vi "AOD Control (FPGA).vi"() -> ()   [LabVIEW 2011]
uses:
  FPGAState.ctl
  AODCalibration.ctl
  CoordinateSettings.ctl
  <vilib>/Platform/TimedLoop/XDataNode/timing_clust.ctl
  <vilib>/Platform/TimedLoop/XDataNode/nitl_modes.ctl
  <vilib>/Platform/TimedLoop/XDataNode/wakeup.ctl
  <vilib>/rvi/eio/common/nirviEmuTemplateMethod_errors.vi
  <vilib>/rvi/interface/RandomDataEmulation/nirviRandomDataFPGAFIFO.vi
  <vilib>/rvi/interface/RandomDataEmulation/niFpgaRandomDataHandleErrors.vi
  <vilib>/Platform/TimedLoop/XDataNode/XDataNode.xnode
  <vilib>/eio/EIONode/EIONode.xnode
  <vilib>/rvi/DataTransferAndStorage/Container/XNode/niFpgaContainer.xnode
  <vilib>/rvi/interface/RandomDataEmulation/nirviRandomDataFpgaReadWriteTemplate.vi
  <vilib>/Platform/TimedLoop/XDataNode/XDNodeRunTimeDep.lvlib
panel:
  out "Debug.Settings":T1 {"YLP_RR" format="%x"; "YLP_FR" format="%x"; "YHP_RR" format="%x"; "YHP_FR" format="%x"; "XLP_RR" format="%x"; "XLP_FR" format="%x"; "XHPstart" format="%x"; "XHPend" format="%x"; "XLPstart" format="%x"; "XLPend" format="%x"; "YHPstart" format="%x"; "YHPend" format="%x"; "YLPstart" format="%x"; "YLPend" format="%x"; "XHP_RR" format="%x"; "XHP_FR" format="%x"}
  out "Raw Full":bool
  in  "Setup.Stop on full":bool
  in  "Setup.BitShift":i16=-10
  in  "Setup.Downsample":u32=1000
  out "Status.Update IO Missing":bool
  out "Status.Last Point":bool
  out "Status.All Samples":bool
  out "Status.Serial error":bool
  out "Status.AcqState":enum16{"Idling", "Acquiring"}(ring)
  out "Status.TemporalChFull":bool
  out "Status.MotionChFull":bool
  out "Status.DownsampleDone":bool
  out "Status.ImChFull":bool
  out "Status.BufferedPoints":i32
  out "Status.State":T2
  out "Status.Initialized":bool
  out "Status.RepNum":u32
  out "Status.OutOfRange":bool
  out "Status.Mode":enum16{"Points", "Volume", "Idle"}(ring)
  out "Status.ScanDone":bool
  out "Status.Armed":bool
  out "Status.ScanUpdateIO":bool
  out "Status.Writing":bool
  out "Status.PointTime":u32
  out "Status.PointNum":u32
  out "Status.Sequencing error":bool
  out "Analog Data":i16[](array[numeric])
  in  "Update IO timeout":u32=40
  out "UpdateIO counter":u32
  in  "AOD.Calibration":T3={"XHP ChirpGain"=1.0, "YHP ChirpGain"=1.0, "XLP ChirpGain"=1.0, "YLP ChirpGain"=1.0}
  in  "AOD.ThrowawaySamples":u16=40
  in  "AOD.LP Center Frequency":u32=858993459 format="%x"
  in  "AOD.HP Center Frequency":u32=805306367 format="%x"
  in  "AOD.Range":u32=214748364 format="%x"
  in  "AOD.BlankSamples":u16=500
  in  "AOD.UpdatesPerPoint":u32=2000
  out "Downsample Counter":u32
  in  "Scan.NumMotionPoints":u32
  in  "Scan.Motion Increment":u32
  in  "Scan.TotalSamples":u32
  in  "Scan.VolumeSettings":T4={"XStart"=0, "XEnd"=0, "XNum"=1, "YStart"=0, "YEnd"=0, "YNum"=1, "ZStart"=0, "ZEnd"=0, "ZNum"=1} {"ZNum" min=1 max=10000; "YNum" min=1 max=10000; "XNum" min=1 max=10000}
  in  "Scan.NumReps":i32=1
  in  "Scan.NumPoints":u32
  out "Scan.Samples":u32
  out "Debug.PMT_Unpacked_backlog":u32
  out "Debug.PMT_Data_backlog":u32
  in  "Debug.FinishedSettingSize":i16=3
  in  "Debug.FinishedSetting":cluster{"Address":u8, "Value":u32}[](array[cluster])=[{"Address"=0, "Value"=246}, {"Address"=4, "Value"=0}, {"Address"=5, "Value"=0}, {"Address"=0, "Value"=0}, {"Address"=0, "Value"=0}] {"Address" format="%x"; "Value" format="%x"}
  in  "Debug.Coordinate":T5
  in  "Debug.SetCoordinate":bool
  out "Debug.AcqDivCount":u32
  out "Debug.PMT_Samples":u32
  out "Debug.MainLoopCount":i32
  in  "Debug.UpdateIO":bool
  out "Debug.PMT Array":i32[](array[numeric])
  in  "Debug.P":bool
  in  "Debug.Point":cluster{"X":i32, "Y":i32, "Z":i32}
  in  "Debug.Write Point":bool
  in  "Control.Points":bool
  in  "Control.Reset":bool
  in  "Control.Abort":bool
  in  "Control.Volume":bool
  in  "Control.Stop":bool
  in  "Comm.P high":u32=10
  in  "Comm.Pause":u32
  in  "Comm.WriteSize":i32
  in  "Comm.Write":cluster{"Address":u8, "Value":u32}[](array[cluster])=[{"Address"=0, "Value"=0}, {"Address"=0, "Value"=0}, {"Address"=0, "Value"=0}, {"Address"=0, "Value"=0}, {"Address"=0, "Value"=0}, {"Address"=0, "Value"=0}, {"Address"=0, "Value"=0}, {"Address"=0, "Value"=0}, {"Address"=0, "Value"=0}, {"Address"=0, "Value"=0}, {"Address"=0, "Value"=0}, {"Address"=0, "Value"=0}, {"Address"=0, "Value"=0}, {"Address"=0, "Value"=0}, {"Address"=0, "Value"=0}, {"Address"=0, "Value"=0}, {"Address"=0, "Value"=0}, {"Address"=0, "Value"=0}, {"Address"=0, "Value"=0}, {"Address"=0, "Value"=0}]
  out "Comm.Written":cluster{"Address":u8, "Value":u32}[](array[cluster])
  out "Comm.WritenCount":i32
  in  "Comm.Write Register":bool
  in  "Comm.SclkDivider":u32=10
  in  "Comm.CommLines":enum16{"1", "2", "4"}(ring)
  out "Comm.Bad Coordinate":bool
  in  "Comm.UpdateIO time":u32=2
  # "TriggerAcq makes this task\n require a trigger from Trig7"
  # "FPGA Control state chart:\n1. Idles\n2. Write series of registers\n3. Receive volume settings or points, \n    arms task, starts  acq clock.  \n4. Clock in first value, waits for Trig7\n5. On Trig7 pulse start task\n6. Pulse update_io, clock point, count\n    downsample number of acq clocks"
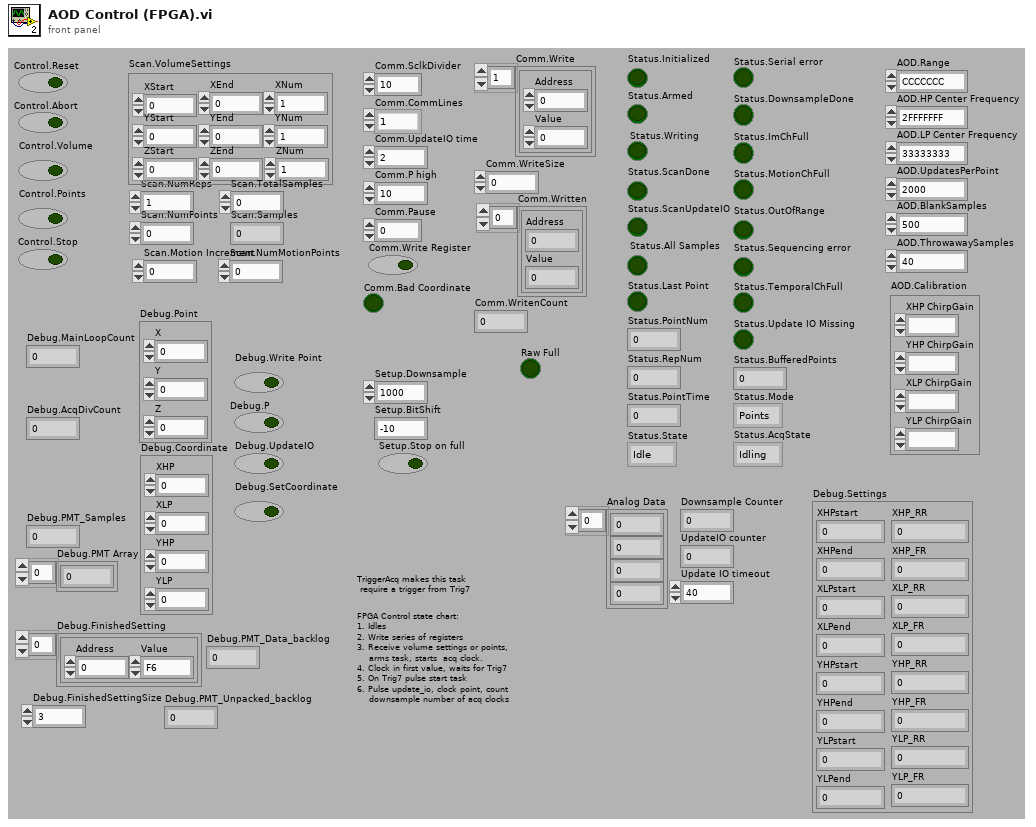
[diagram p1: front panel]
types:
  T1 = typedef "CoordinateSettings.ctl" = cluster{"XHPstart":u32, "XHPend":u32, "XLPstart":u32, "XLPend":u32, "YHPstart":u32, "YHPend":u32, "YLPstart":u32, "YLPend":u32, "XHP_RR":u32, "XHP_FR":u32, "XLP_FR":u32, "XLP_RR":u32, "YHP_FR":u32, "YHP_RR":u32, "YLP_FR":u32, "YLP_RR":u32}
  T2 = typedef "FPGAState.ctl" = enum16{"Idle", "Arm Scan", "Scan", "End Scan"}
  T3 = typedef "AODCalibration.ctl" = cluster{"XHP ChirpGain":fxp<+/-,16,2>, "YHP ChirpGain":fxp<+/-,16,2>, "XLP ChirpGain":fxp<+/-,16,2>, "YLP ChirpGain":fxp<+/-,16,2>}
  T4 = cluster{"XStart":i32, "XEnd":i32, "XNum":i32, "YStart":i32, "YEnd":i32, "YNum":i32, "ZStart":i32, "ZEnd":i32, "ZNum":i32}
  T5 = cluster{"XHP":i32, "XLP":i32, "YHP":i32, "YLP":i32}
  T6 = cluster{"Scan mode":enum16{"Points", "Volume", "Idle"}, "NumPoints":u32, "NumReps":u32, "Motion Increment":u32, "NumMotionPoints":u32, "VolumeSettings":cluster{"XStart":i32, "XEnd":i32, "XNum":i32, "YStart":i32, "YEnd":i32, "YNum":i32, "ZStart":i32, "ZEnd":i32, "ZNum":i32}}
  T7 = typedef "XDNodeRunTimeDep.lvlib/timing_clust.ctl" = cluster{"Expected End [f-1]":u64, "Actual End [f-1]":u64, "Finished Late? [f-1]":bool, "Expected End [i-1]":u64, "Actual End [i-1]":u64, "Finished Late? [i-1]":bool, "Expected Start [i]":u64, "Actual Start [i]":u64, "Expected Start [f]":u64, "Actual Start [f]":u64, "Source Name":string, "Structure Name":string, "Period":i64, "Deadline":i64, "Offset":i64, "Start":i64, "Priority":i32, "Timeout":i32, "Mode":T8, "Wakeup Reason":T9, "Error":errorcluster, "Source Type":string, "Secondary Source Type":string, "Global End Time":u64, "Global Start Time":u64, "Frame Duration":u64, "Iteration Duration":u64, "Assigned CPU":i32, "I/O Scan Engine Mode":u32}
  T8 = typedef "XDNodeRunTimeDep.lvlib/nitl_modes.ctl" = enum32{"No Change", "Process missed periods, maintain original phase", "Discard missed periods, maintain original phase", "Process missed periods, ignore original phase", "Discard missed periods, ignore original phase"}
  T9 = typedef "XDNodeRunTimeDep.lvlib/wakeup.ctl" = enum32{"Normal", "Aborted", "Asynchronous wakeup", "Timing source error", "Timed loop error", "Timeout"}
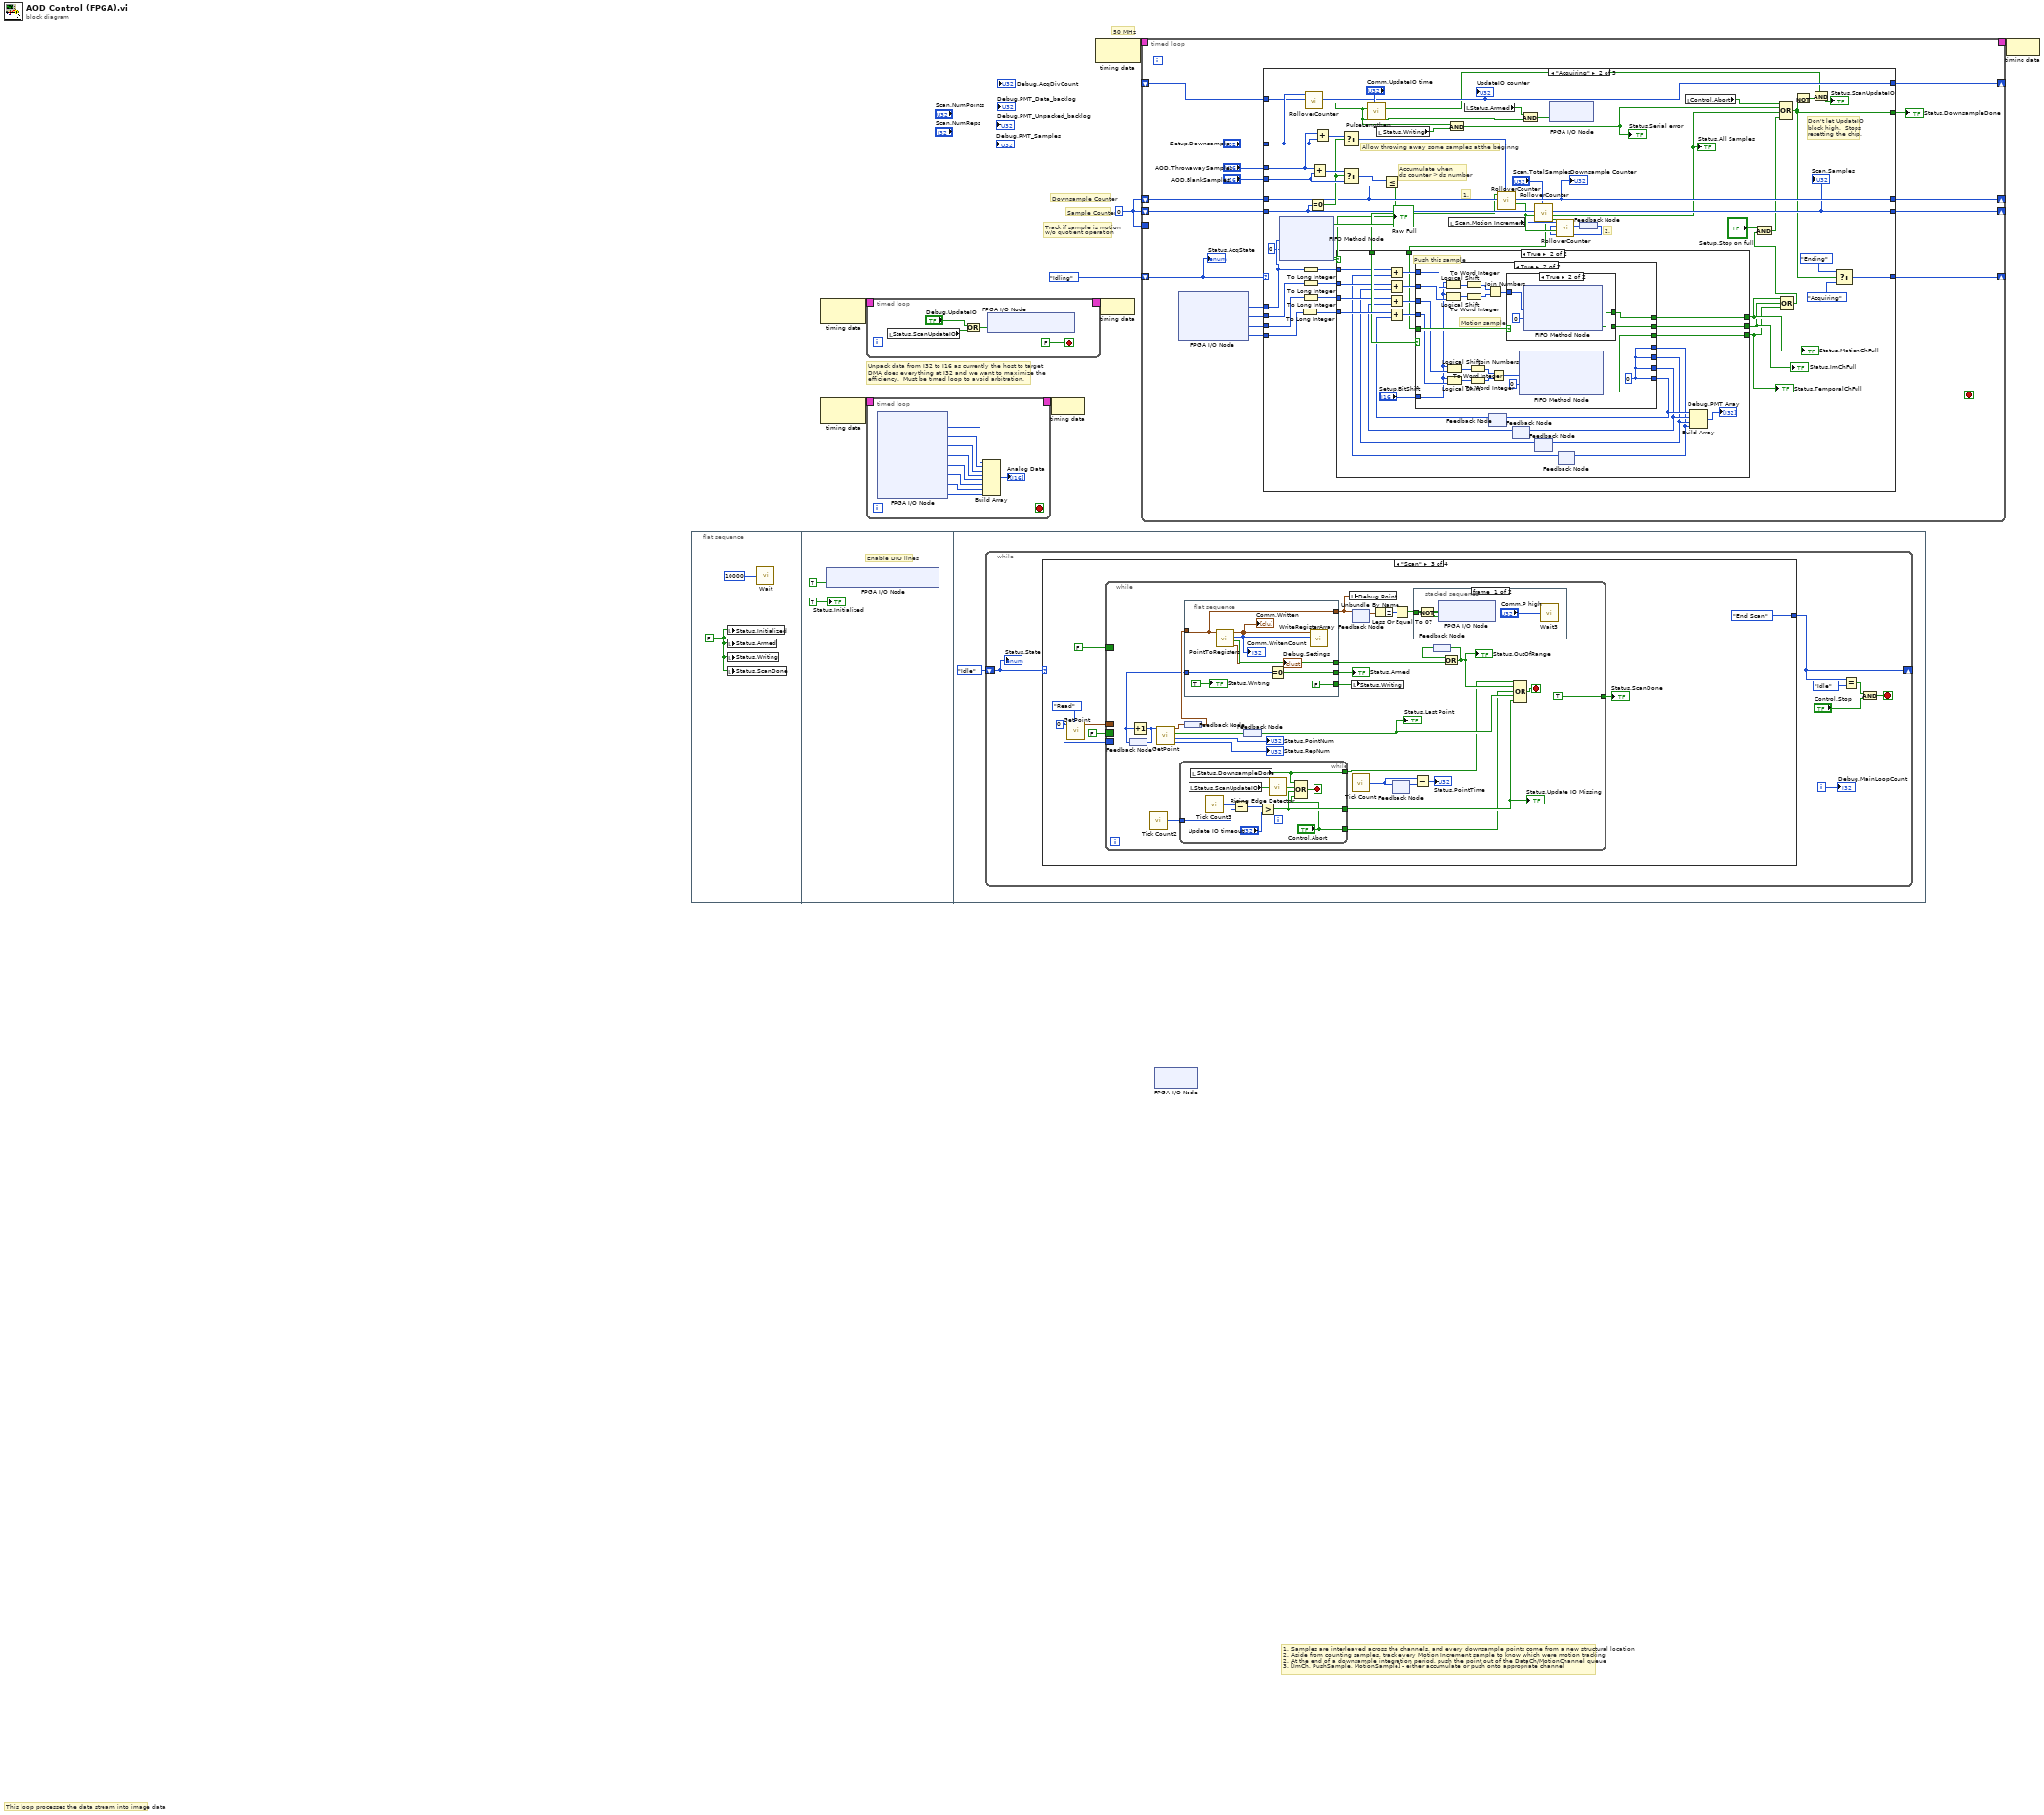
[diagram p0: block diagram]
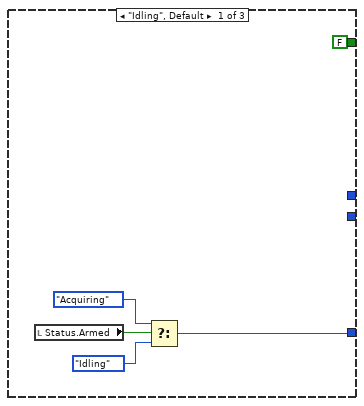
[diagram p2: hidden frame]
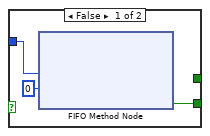
[diagram p5: hidden frame]
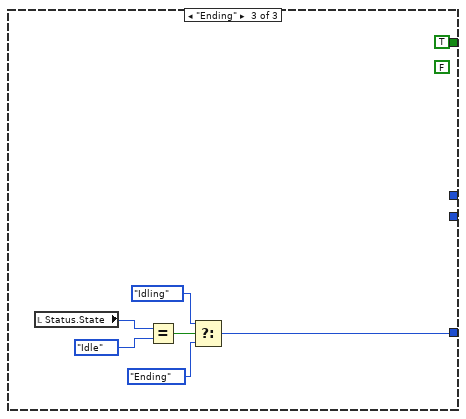
[diagram p6: hidden frame]
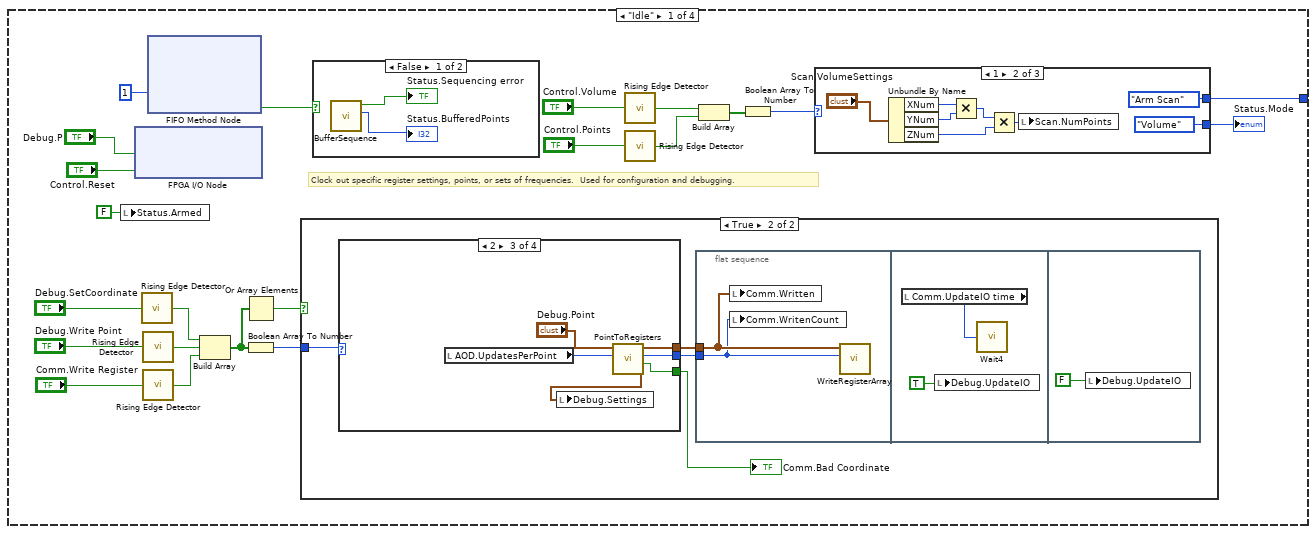
[diagram p7: hidden frame]
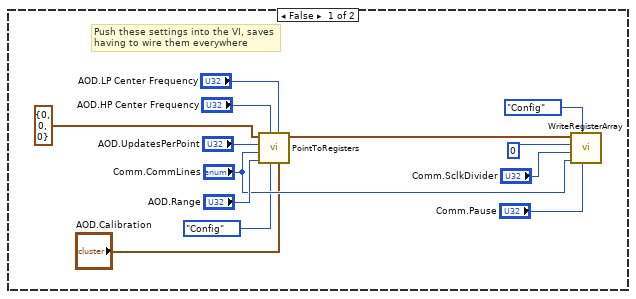
[diagram p9: hidden frame]
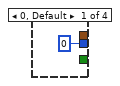
[diagram p10: hidden frame]
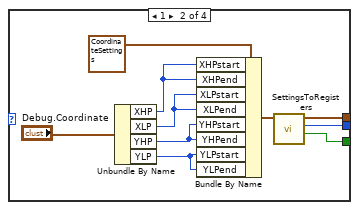
[diagram p11: hidden frame]
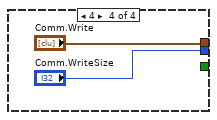
[diagram p12: hidden frame]
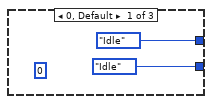
[diagram p13: hidden frame]
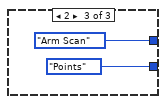
[diagram p14: hidden frame]
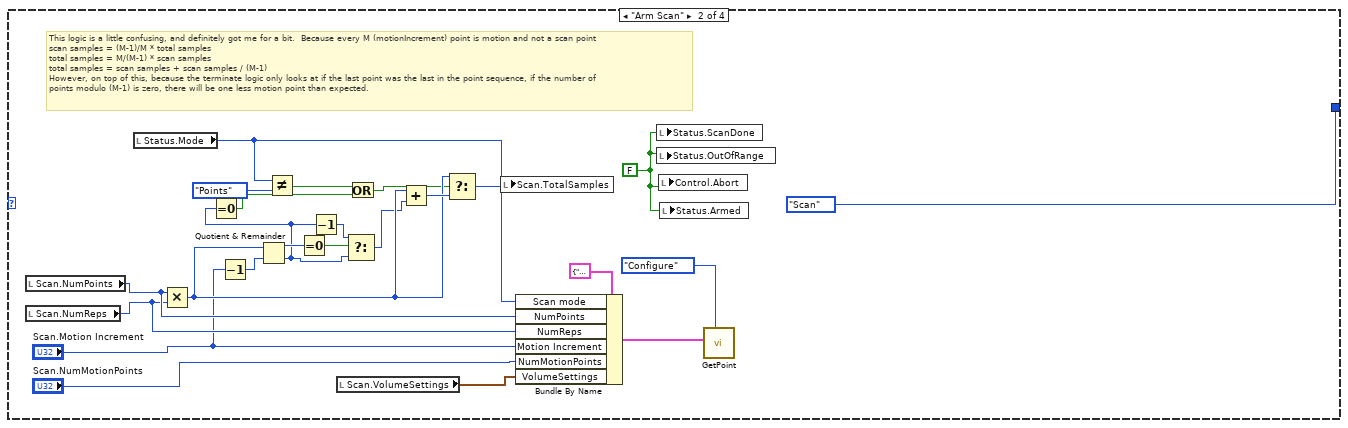
[diagram p15: hidden frame]
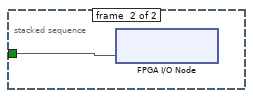
[diagram p16: hidden frame]
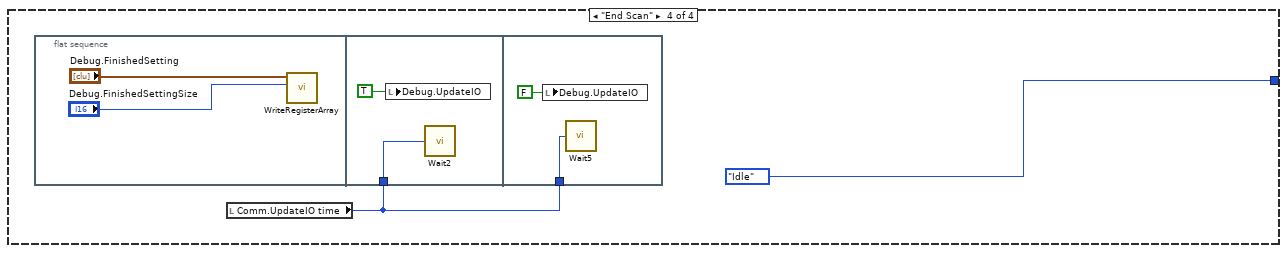
[diagram p17: hidden frame]
diagram:
  w6 = u32 0
  # "Downsample Counter"
  # "Sample Counter"
  # "Track if sample is motion\nw/o quotient operation"
  # "50 MHz"
  # "Unpack data from I32 to I16 as currently the host to target\nDMA does everything at I32 and we want to maximize the\nefficiency.  Must be timed loop to avoid arbitration."
  # "1. Samples are interleaved across the channels, and every downsample points come from a new structural location\n2. Aside from counting samples, track every Motion Increment sample to know which were motion tracking\n2. At the end of a downsample integration period, push the point out of the DataCh/MotionChannel queue\n3. [ImCh, PushSample, MotionSample] - either accumulate or push onto appropriate channel"
  # "This loop processes the data stream into image data"
  n1 = flat-sequence {
    frame #0 {
      w9 = FALSE
      n2 = local write "Status.Initialized"(w9) -> ()
      n3 = local write "Status.Armed"(w9) -> ()
      n4 = local write "Status.Writing"(w9) -> ()
      n5 = local write "Status.ScanDone"(w9) -> ()
      n6 = call "Wait"("Count(uSec)"=u32 10000) -> ()  [unwired: 1 out]
    }
    frame #1 {
      # "Enable DIO lines"
      n7 = xnode "FPGA I/O Node"("IO Module\\Digital Output Enable"=TRUE ("IO Module\\DDCA_DIO0-7_WE")) -> ()  [unwired: 1 in, 1 out]
      "Status.Initialized" <- TRUE ("Status.Initialized")
    }
    frame #2 {
      n8 = while {
        shift-right: [w19] -> _
        shift-left: FPGAState."Idle" ("Ring") -> [w14]
        i -> [w20]
        stop <- w16 stop-if-true
        n9 = case shown="\"Scan\"" w14 {
          tunnel: [w41 FPGAState."Scan" ("Ring") FPGAState."End Scan" ("Ring") FPGAState."Idle" ("Enum")] -> w19
          frame "Idle" {
            # "Clock out specific register settings, points, or sets of frequencies.  Used for configuration and debugging."
            n10 = local write "Status.Armed"(FALSE ("Status.Armed")) -> ()
            n11 = xnode "FPGA I/O Node"("IO Module\\P"="Debug.P", "IO Module\\RESET"="Control.Reset") -> ()  [unwired: 2 in, 2 out]
            n12 = call "Rising Edge Detector.vi"("Signal In"="Debug.SetCoordinate") -> ("Edge Detected?"=w34:bool)
            n13 = call "Rising Edge Detector.vi"("Signal In"="Debug.Write Point") -> ("Edge Detected?"=w33:bool)
            n14 = call "Rising Edge Detector.vi"("Signal In"="Comm.Write Register") -> ("Edge Detected?"=w28:bool)
            n15 = xnode ("FIFO Method Node")("Timeout"=1) -> ("Timed Out?"=w27:bool)  [unwired: 1 in, 2 out]
            n16 = Build Array(w34, w33, w28) -> (w32:bool[])
            n17 = Or Array Elements(Boolean array=w32) -> (logical OR=w31:bool)
            n18 = Boolean Array To Number(Boolean array=w32) -> (number=w30:u8)
            n19 = case shown="True" w31 {
              tunnel: w30 -> [_ w61]
              frame False {
                # "Push these settings into the VI, saves \nhaving to wire them everywhere"
                n20 = call "PointToRegisters.vi"("Calibration"="AOD.Calibration", "LP Center Frequency"="AOD.LP Center Frequency", "Mode"=enum16{"Normal", "Config"}."Config", "HP Center Frequency"="AOD.HP Center Frequency", "Range"="AOD.Range", "WriteSize"="Comm.CommLines", "UpdatesPerPoint"="AOD.UpdatesPerPoint", "Point"=cluster{"X":i32, "Y":i32, "Z":i32} {"X"=0, "Y"=0, "Z"=0}) -> ("Register Writes"=w45:cluster{"Address":u8, "Value":u32}[])  [unwired: 3 out]
                n21 = call "WriteRegisterArray.vi"("Pause"="Comm.Pause", "Mode"=enum16{"Normal", "Config"}."Config", "WriteSize"="Comm.CommLines", "SclkDivider"="Comm.SclkDivider", "NumReg"=i16 0, "Register  Values"=w45) -> ()  [unwired: 6 in]
              }
              frame True {
                n22 = case shown="2" w61 {
                  tunnel: [_ w71 w82 "Comm.Write"] -> w59
                  tunnel: [i16 0 ("WriteLength") w70 w81 "Comm.WriteSize"] -> w60
                  tunnel: [_ w69 w80 _] -> w58
                  frame 0, Default {
                  }
                  frame 1 {
                    n23 = Unbundle By Name("Debug.Coordinate") -> ("XHP"=w77:i32, "XLP"=w76:i32, "YHP"=w75:i32, "YLP"=w74:i32)
                    n24 = Bundle By Name(cluster=T1 {"XHPstart"=0, "XHPend"=0, "XLPstart"=0, "XLPend"=0, "YHPstart"=0, "YHPend"=0, "YLPstart"=0, "YLPend"=0, "XHP_RR"=0, "XHP_FR"=0, "XLP_FR"=0, "XLP_RR"=0, "YHP_FR"=0, "YHP_RR"=0, "YLP_FR"=0, "YLP_RR"=0} ("settings"), "XHPstart"=w77, "XHPend"=w77, "XLPstart"=w76, "XLPend"=w76, "YHPstart"=w75, "YHPend"=w75, "YLPstart"=w74, "YLPend"=w74) -> (w73:T1)
                    n25 = call "SettingsToRegisters.vi"("coordinates"=w73) -> ("OutOfRange"=w69:bool, "size(s)"=w70:i32, "Register Writes"=w71:cluster{"Address":u8, "Value":u32}[])  [unwired: 8 in]
                  }
                  frame 2 {
                    n26 = local read "AOD.UpdatesPerPoint"() -> (w83:u32)
                    n27 = call "PointToRegisters.vi"("UpdatesPerPoint"=w83, "Point"="Debug.Point") -> ("settings"=w78:T1, "OutOfRange"=w80:bool, "Number Registers"=w81:i16, "Register Writes"=w82:cluster{"Address":u8, "Value":u32}[])  [unwired: 6 in]
                    n28 = local write "Debug.Settings"(w78) -> ()
                  }
                  frame 4 {
                  }
                }
                "Comm.Bad Coordinate" <- w58
                n29 = flat-sequence {
                  tunnel: w60 -> [w62]
                  tunnel: w59 -> [w63]
                  frame #0 {
                    n30 = local write "Comm.Written"(w63) -> ()
                    n31 = local write "Comm.WritenCount"(w62) -> ()
                    n32 = call "WriteRegisterArray.vi"("NumReg"=w62, "Register  Values"=w63) -> ()  [unwired: 10 in]
                  }
                  frame #1 {
                    n33 = local read "Comm.UpdateIO time"() -> (w65:u32)
                    n34 = local write "Debug.UpdateIO"(TRUE ("UpdateIO")) -> ()
                    n35 = call "Wait4"("Count(Ticks)"=w65) -> ()  [unwired: 1 out]
                  }
                  frame #2 {
                    n36 = local write "Debug.UpdateIO"(FALSE ("UpdateIO")) -> ()
                  }
                }
              }
            }
            n37 = case shown="False" w27 {
              frame False {
                n38 = call "BufferSequence.vi"() -> ("NumPoints"=→"Status.BufferedPoints":i32, "Sequencing error"=→"Status.Sequencing error":bool)  [unwired: 10 in]
              }
              frame True {
              }
            }
            n39 = call "Rising Edge Detector.vi"("Signal In"="Control.Volume") -> ("Edge Detected?"=w25:bool)
            n40 = call "Rising Edge Detector.vi"("Signal In"="Control.Points") -> ("Edge Detected?"=w24:bool)
            n41 = Build Array(w25, w24) -> (w23:bool[])
            n42 = Boolean Array To Number(Boolean array=w23) -> (number=w22:u8)
            n43 = case shown="1" w22 {
              tunnel: [FPGAState."Idle" ("Ring") FPGAState."Arm Scan" ("Ring") FPGAState."Arm Scan" ("Ring")] -> w41
              tunnel: [enum16{"Points", "Volume", "Idle"}."Idle" ("Mode") enum16{"Points", "Volume", "Idle"}."Volume" ("Mode") enum16{"Points", "Volume", "Idle"}."Points" ("Mode")] -> w38
              frame 0, Default {
                (unwired) 0 ("BufferedPoints")
              }
              frame 1 {
                n44 = Unbundle By Name("Scan.VolumeSettings") -> ("XNum"=w93:i32, "YNum"=w92:i32, "ZNum"=w90:i32)
                n45 = Multiply(x=w93, y=w92) -> (x*y=w91:i32)
                n46 = Multiply(x=w91, y=w90) -> (x*y=w88:i32)
                n47 = local write "Scan.NumPoints"(w88) -> ()
              }
              frame 2 {
              }
            }
            "Status.Mode" <- w38
          }
          frame "Arm Scan" {
            w98 = FALSE ("ScanDone")
            # "This logic is a little confusing, and definitely got me for a bit.  Because every M (motionIncrement) point is motion and not a scan point\nscan samples = (M-1)/M * total samples\ntotal samples = M/(M-1) * scan samples\ntotal samples = scan samples + scan samples / (M-1)\nHowever, on top of this, because the terminate logic only looks at if the last point was the last in the point sequence, if the number of\npoints modulo (M-1) is zero, there will be one less motion point than expected."
            n48 = local read "Scan.NumPoints"() -> (w116:u32)
            n49 = local read "Scan.NumReps"() -> (w115:i32)
            n50 = local read "Status.Mode"() -> (w113:enum16{"Points", "Volume", "Idle"})
            n51 = Multiply(x=w116, y=w115) -> (x*y=w109:u32)
            n52 = Decrement(x="Scan.Motion Increment") -> (x-1=w107:u32)
            n53 = Quotient & Remainder(x=w109, y=w107) -> (x-y*floor(x/y)=w106:u32, floor(x/y)=w100:u32)
            n54 = Equal To 0?(x=w100) -> (x = 0?=w105:bool)
            n55 = Not Equal?(x=w113, y=enum16{"Points", "Volume", "Idle"}."Points") -> (x != y?=w104:bool)
            n56 = Equal To 0?(x=w106) -> (x = 0?=w102:bool)
            n57 = Decrement(x=w100) -> (x-1=w101:u32)
            n58 = local read "Scan.VolumeSettings"() -> (w117:T4)
            n59 = Select(t=w101, s=w102, f=w100) -> (s? t:f=w99:u32)
            n60 = Or(x=w104, y=w105) -> (x .or. y?=w103:bool)
            n61 = Add(x=w109, y=w99) -> (x+y=w111:u32)
            n62 = Select(t=w109, s=w103, f=w111) -> (s? t:f=w110:u32)
            n63 = local write "Scan.TotalSamples"(w110) -> ()
            n64 = Bundle By Name(cluster=T6 {"Scan mode"=enum."Points", "NumPoints"=0, "NumReps"=0, "Motion Increment"=0, "NumMotionPoints"=0, "VolumeSettings"={"XStart"=0, "XEnd"=0, "XNum"=1, "YStart"=0, "YEnd"=0, "YNum"=1, "ZStart"=0, "ZEnd"=0, "ZNum"=1}} ("Settings"), "Scan mode"=w113, "NumPoints"=w116, "NumReps"=w115, "Motion Increment"="Scan.Motion Increment", "NumMotionPoints"="Scan.NumMotionPoints", "VolumeSettings"=w117) -> (w118:T6)
            n65 = local write "Status.ScanDone"(w98) -> ()
            n66 = local write "Status.OutOfRange"(w98) -> ()
            n67 = local write "Control.Abort"(w98) -> ()
            n68 = local write "Status.Armed"(w98) -> ()
            n69 = call "GetPoint.vi"("Mode"=enum16{"Read", "Configure"}."Configure", "Settings"=w118) -> ()  [unwired: 6 in, 4 out]
          }
          frame "Scan" {
            w123 = u32 0 ("Sample Number")
            n70 = call "GetPoint.vi"("Mode"=enum16{"Read", "Configure"}."Read", "Sample Number"=w123) -> ("Point"=w125:cluster{"X":i32, "Y":i32, "Z":i32})  [unwired: 6 in, 3 out]
            n71 = while {
              border: FALSE ("OutOfRange") -> [_]
              tunnel: [TRUE] -> w126
              border: w125 -> [_]
              border: FALSE ("Done") -> [_]
              border: w123 -> [_]
              stop <- w148 stop-if-true
              n72 = feedback #1() -> (w132:u32)
              n73 = Increment(x=w132) -> (x+1=w140:u32)
              n74 = feedback-in #1(w140) -> ()
              n75 = call "Tick Count2"() -> ("Tick Count(uSec)"=w134:u32)
              n76 = call "GetPoint.vi"("Sample Number"=w140) -> ("RepNum"=→"Status.RepNum":u32, "Point Num"=→"Status.PointNum":u32, "Done"=w141:bool, "Point"=w143:cluster{"X":i32, "Y":i32, "Z":i32})  [unwired: 7 in]
              n77 = while {
                tunnel: w134 -> [w162]
                tunnel: [w158] -> w133
                tunnel: ["Control.Abort"] -> w130
                tunnel: [w155] -> w129
                stop <- w159 stop-if-true
                n78 = local read "Status.ScanUpdateIO"() -> (w164:bool)
                n79 = local read "Status.DownsampleDone"() -> (w155:bool)
                n80 = call "Tick Count3"() -> ("Tick Count(uSec)"=w163:u32)
                n81 = Subtract(x=w163, y=w162) -> (x-y=w161:u32)
                n82 = Greater?(x=w161, y="Update IO timeout") -> (0:w158:bool)
                n83 = call "Rising Edge Detector.vi"("Signal In"=w164) -> ("Edge Detected?"=w160:bool)
                n84 = Compound Arithmetic op=OR(w155, w160, w158, "Control.Abort") -> (w159:bool)
              }
              "Status.Update IO Missing" <- w133
              n85 = flat-sequence {
                tunnel: w142 -> [w172]
                tunnel: [FALSE] -> w147
                tunnel: [w170] -> w135
                tunnel: [w175] -> w145
                tunnel: [w172] -> w139
                tunnel: w132 -> [w171]
                frame #0 {
                  n86 = call "PointToRegisters.vi"("Point"=w172) -> ("settings"=→"Debug.Settings":T1, "OutOfRange"=w175:bool, "Number Registers"=w173:i16, "Register Writes"=w174:cluster{"Address":u8, "Value":u32}[])  [unwired: 7 in]
                  "Comm.Written" <- w174
                  "Comm.WritenCount" <- w173
                  n87 = Equal To 0?(x=w171) -> (x = 0?=w170:bool)
                  n88 = call "WriteRegisterArray.vi"("NumReg"=w173, "Register  Values"=w174) -> ()  [unwired: 10 in]
                  "Status.Writing" <- TRUE ("Writing")
                }
              }
              n89 = feedback-in #2(w143) -> ()
              n90 = feedback #2() -> (w142:cluster{"X":i32, "Y":i32, "Z":i32})
              n91 = feedback-in #3(w141) -> ()
              n92 = feedback #3() -> (w136:bool)
              "Status.Last Point" <- w136
              n93 = local write "Debug.Point"(w139) -> ()
              n94 = local write "Status.Writing"(w147) -> ()
              n95 = feedback-in #4(w139) -> ()
              n96 = feedback #4() -> (w152:cluster{"X":i32, "Y":i32, "Z":i32})  [unwired: 1 in]
              n97 = call "Tick Count"() -> ("Tick Count(Ticks)"=w150:u32)
              n98 = Unbundle By Name(w152) -> ("Z"=w153:i32)
              n99 = feedback-in #5(w150) -> ()
              n100 = feedback #5() -> (w149:u32)  [unwired: 1 in]
              n101 = Less Or Equal To 0?(x=w153) -> (x <= 0?=w151:bool)
              n102 = stacked-sequence {
                tunnel: w151 -> [w166 w168]
                frame #0 {
                  n103 = Not(x=w166) -> (.not. x?=w165:bool)
                  n104 = xnode "FPGA I/O Node"("IO Module\\P"=w165) -> ()  [unwired: 1 in, 1 out]
                  n105 = call "Wait3"("Count(Ticks)"="Comm.P high") -> ()  [unwired: 1 out]
                }
                frame #1 {
                  n106 = xnode "FPGA I/O Node"("IO Module\\P"=w168) -> ()  [unwired: 1 in, 1 out]
                }
              }
              n107 = Subtract(x=w150, y=w149) -> (x-y=→"Status.PointTime":u32)
              n108 = feedback #6() -> (w146:bool)
              n109 = Or(x=w146, y=w145) -> (x .or. y?=w131:bool)
              "Status.OutOfRange" <- w131
              n110 = feedback-in #6(w131) -> ()
              n111 = Compound Arithmetic op=OR(w129, w131, w130, w136, w133) -> (w148:bool)
              "Status.Armed" <- w135
            }
            "Status.ScanDone" <- w126
          }
          frame "End Scan" {
            n112 = flat-sequence {
              tunnel: w178 -> [w182]
              tunnel: w178 -> [w184]
              frame #0 {
                n113 = call "WriteRegisterArray.vi"("NumReg"="Debug.FinishedSettingSize", "Register  Values"="Debug.FinishedSetting") -> ()  [unwired: 10 in]
              }
              frame #1 {
                n114 = local write "Debug.UpdateIO"(TRUE ("Debug.UpdateIO")) -> ()
                n115 = call "Wait2"("Count(Ticks)"=w182) -> ()  [unwired: 1 out]
              }
              frame #2 {
                n116 = local write "Debug.UpdateIO"(FALSE ("Debug.UpdateIO")) -> ()
                n117 = call "Wait5"("Count(Ticks)"=w184) -> ()  [unwired: 1 out]
              }
            }
            n118 = local read "Comm.UpdateIO time"() -> (w178:u32)
          }
        }
        n119 = Equal?(x=w19, y=FPGAState."Idle" ("Ring")) -> (x = y?=w18:bool)
        n120 = And(x=w18, y="Control.Stop") -> (x .and. y?=w16:bool)
        "Debug.MainLoopCount" <- w20
        "Status.State" <- w14
      }
    }
  }
  n121 = node-c288() -> (w4:T7)  [unwired: 1 in]
  n122 = node-c288() -> (w2:T7)  [unwired: 1 in]
  n123 = timed-loop {
    timing: w4 -> [_]
    timing-out: [_] -> w3
    stop <- FALSE stop-if-true
    n124 = local read "Status.ScanUpdateIO"() -> (w188:bool)
    n125 = Or(x="Debug.UpdateIO", y=w188) -> (x .or. y?=w186:bool)
    n126 = xnode "FPGA I/O Node"("IO Module\\UPDATE_IO"=w186) -> ()  [unwired: 1 in, 1 out]
  }
  n127 = timed-loop {
    timing: w2 -> [_]
    timing-out: [_] -> w1
    stop <- _ stop-if-true
    n128 = xnode "FPGA I/O Node"() -> ("IO Module\\AI A0"=w196:i16, "IO Module\\AI A1"=w195:i16, "IO Module\\AI A2"=w194:i16, "IO Module\\AI A3"=w193:i16, "IO Module\\AI A4"=w200:i16, "IO Module\\AI A5"=w199:i16, "IO Module\\AI A6"=w198:i16, "IO Module\\AI A7"=w197:i16)  [unwired: 8 in, 8 out]
    n129 = Build Array(w196, w195, w194, w193, w200, w199, w198, w197) -> (→"Analog Data":i16[])
  }
  n130 = node-c288(w1) -> ()
  n131 = node-c288() -> (w8:T7)  [unwired: 1 in]
  n132 = node-c288(w3) -> ()
  n133 = timed-loop {
    shift-right: [w216] -> _
    shift-left: w6 -> [w218]
    timing: w8 -> [_]
    timing-out: [_] -> w7
    shift-right: [w217] -> _
    shift-left: w6 -> [w215]
    border: w6 -> [_]
    shift-right: [w209] -> _
    shift-left: enum16{"Idling", "Acquiring", "Ending"}."Idling" -> [w214]
    shift-right: [w204] -> _
    shift-left: _ -> [w203]
    stop <- _ stop-if-true
    n134 = xnode "FPGA I/O Node"() -> ("IO Module\\AI A0"=w213:i16, "IO Module\\AI A1"=w212:i16, "IO Module\\AI A2"=w211:i16, "IO Module\\AI A3"=w210:i16)  [unwired: 4 in, 4 out]
    n135 = case shown="\"Acquiring\"" w214 {
      tunnel: "AOD.BlankSamples" -> [_ w276 _]
      tunnel: "Setup.Downsample" -> [_ w246 _]
      tunnel: w218 -> [_ w273 _]
      tunnel: [_ w272 _] -> w217
      tunnel: [_ w270 _] -> w216
      tunnel: w215 -> [_ w267 _]
      tunnel: "AOD.ThrowawaySamples" -> [_ w266 _]
      tunnel: w213 -> [_ w230 _]
      tunnel: w212 -> [_ w253 _]
      tunnel: w211 -> [_ w252 _]
      tunnel: w210 -> [_ w251 _]
      tunnel: [w223 w250 w333] -> w209
      tunnel: [FALSE w227 TRUE] -> w208
      tunnel: [_ w247 _] -> w204
      tunnel: w203 -> [_ w245 _]
      frame "Idling", Default {
        n136 = local read "Status.Armed"() -> (w219:bool)
        n137 = Select(t=enum16{"Idling", "Acquiring"}."Acquiring" ("AcqState"), s=w219, f=enum16{"Idling", "Acquiring"}."Idling" ("AcqState")) -> (s? t:f=w223:enum16{"Idling", "Acquiring"})
      }
      frame "Acquiring" {
        # "Don't let UpdateIO\nblock high.  Stops \nresetting the chip."
        # "Allow throwing away some samples at the beginng"
        # "2."
        # "1."
        # "Accumulate when \nds counter > ds number"
        n138 = xnode ("FIFO Method Node")("Element"=w230, "Timeout"=0) -> ("Timed Out?"=→"Raw Full":bool)  [unwired: 1 in, 1 out]
        n139 = To Long Integer(number=w251) -> (32bit integer=w265:i32)
        n140 = To Long Integer(number=w230) -> (32bit integer=w262:i32)
        n141 = To Long Integer(number=w253) -> (32bit integer=w263:i32)
        n142 = To Long Integer(number=w252) -> (32bit integer=w264:i32)
        n143 = call "RolloverCounter.vi"("RolloverNum"=w246, "In"=w245) -> ("Rollover"=w231:bool, "Count"=w247:u32)  [unwired: 7 in, 1 out]
        "UpdateIO counter" <- w247
        n144 = Equal To 0?(x=w273) -> (x = 0?=w268:bool)
        n145 = Add(x=w266, y=w276) -> (x+y=w275:u16)
        n146 = Add(x=w266, y=w246) -> (x+y=w274:u32)
        n147 = Select(t=w274, s=w268, f=w246) -> (s? t:f=w271:u32)
        n148 = Select(t=w275, s=w268, f=w276) -> (s? t:f=w269:u16)
        n149 = call "PulseLengthen.vi"("Lengthen"="Comm.UpdateIO time", "Pulse"=w231) -> ("Lengthened"=w225:bool)  [unwired: 9 in]
        n150 = local read "Status.Writing"() -> (w244:bool)
        n151 = Less Or Equal?(x=w269, y=w267) -> (x <= y?=w254:bool)
        n152 = And(x=w231, y=w244) -> (x .and. y?=w237:bool)
        "Status.Serial error" <- w237
        n153 = local read "Scan.Motion Increment"() -> (w257:u32)
        n154 = local read "Status.Armed"() -> (w232:bool)
        n155 = call "RolloverCounter.vi"("RolloverNum"=w271, "In"=w267) -> ("Rollover"=w260:bool, "Count"=w272:u32, "Last"=w248:bool)  [unwired: 7 in]
        "Downsample Counter" <- w272
        n156 = And(x=w232, y=w231) -> (x .and. y?=w233:bool)
        n157 = call "RolloverCounter.vi"("RolloverNum"="Scan.TotalSamples", "Increment"=w260, "In"=w273) -> ("Rollover"=w238:bool, "Count"=w270:u32)  [unwired: 6 in, 1 out]
        "Scan.Samples" <- w270
        "Status.All Samples" <- w238
        n158 = xnode "FPGA I/O Node"("TRIG5"=w233) -> ()  [unwired: 1 in, 1 out]
        n159 = feedback #7() -> (w258:u32)
        n160 = call "RolloverCounter.vi"("RolloverNum"=w257, "Increment"=w260, "In"=w258) -> ("Count"=w259:u32, "Last"=w256:bool)  [unwired: 6 in, 1 out]
        n161 = case shown="True" w254 {
          tunnel: w262 -> [_ w288]
          tunnel: w263 -> [_ w292]
          tunnel: w264 -> [_ w295]
          tunnel: w265 -> [_ w299]
          tunnel: w248 -> [_ w298]
          tunnel: w256 -> [_ w286]
          tunnel: [_ w279] -> w241
          tunnel: [_ w278] -> w240
          tunnel: [_ w277] -> w239
          frame False {
          }
          frame True {
            # "Push this sample"
            n162 = feedback #8() -> (w296:i32)  [unwired: 1 in]
            n163 = Add(x=w299, y=w296) -> (x+y=w297:i32)
            n164 = feedback #9() -> (w293:i32)  [unwired: 1 in]
            n165 = Add(x=w295, y=w293) -> (x+y=w294:i32)
            n166 = feedback #10() -> (w290:i32)  [unwired: 1 in]
            n167 = Add(x=w292, y=w290) -> (x+y=w291:i32)
            n168 = feedback #11() -> (w287:i32)  [unwired: 1 in]
            n169 = Add(x=w288, y=w287) -> (x+y=w289:i32)
            n170 = case shown="True" w298 {
              tunnel: w297 -> [w303 w319]
              tunnel: [w303 w324] -> w284
              tunnel: [w302 w324] -> w283
              tunnel: w294 -> [w302 w320]
              tunnel: w291 -> [w301 w309]
              tunnel: [w301 w324] -> w282
              tunnel: w289 -> [w300 w308]
              tunnel: [w300 w324] -> w281
              tunnel: w286 -> [_ w321]
              tunnel: "Setup.BitShift" -> [_ w307]
              tunnel: [_ w306] -> w279
              tunnel: [_ w305] -> w278
              tunnel: [_ w304] -> w277
              frame False {
                # "Blanking.  Could also loop zeros and\naccumulate in here later to clean up \ncode"
              }
              frame True {
                w324 = i16 0
                # "Motion sample"
                n171 = Logical Shift(y=w307, x=w308) -> (x << y=w314:i32)
                n172 = Logical Shift(y=w307, x=w309) -> (x << y=w313:i32)
                n173 = Logical Shift(y=w307, x=w320) -> (x << y=w318:i32)
                n174 = Logical Shift(y=w307, x=w319) -> (x << y=w317:i32)
                n175 = To Word Integer(number=w314) -> (16bit integer=w312:i16)
                n176 = To Word Integer(number=w313) -> (16bit integer=w311:i16)
                n177 = To Word Integer(number=w318) -> (16bit integer=w316:i16)
                n178 = To Word Integer(number=w317) -> (16bit integer=w315:i16)
                n179 = Join Numbers(hi=w312, lo=w311) -> ((hi.lo)=w310:u32)
                n180 = Join Numbers(hi=w316, lo=w315) -> ((hi.lo)=w322:u32)
                n181 = case shown="True" w321 {
                  tunnel: w310 -> [w327 w330]
                  tunnel: [_ w328] -> w306
                  tunnel: [w325 _] -> w305
                  frame False {
                    n182 = xnode ("FIFO Method Node")("Element"=w327, "Timeout"=0) -> ("Timed Out?"=w325:bool)  [unwired: 1 in, 1 out]
                  }
                  frame True {
                    n183 = xnode ("FIFO Method Node")("Element"=w330, "Timeout"=0) -> ("Timed Out?"=w328:bool)  [unwired: 1 in, 1 out]
                  }
                }
                n184 = xnode ("FIFO Method Node")("Element"=w322, "Timeout"=0) -> ("Timed Out?"=w304:bool)  [unwired: 1 in, 1 out]
              }
            }
            n185 = feedback-in #8(w284) -> ()
            n186 = feedback-in #9(w283) -> ()
            n187 = feedback-in #10(w282) -> ()
            n188 = feedback-in #11(w281) -> ()
            n189 = Build Array(w284, w283, w282, w281) -> (→"Debug.PMT Array":i32[])
          }
        }
        "Status.TemporalChFull" <- w239
        "Status.ImChFull" <- w240
        "Status.MotionChFull" <- w241
        n190 = feedback-in #7(w259) -> ()
        n191 = local read "Control.Abort"() -> (w255:bool)
        n192 = Compound Arithmetic op=OR(w241, w240, w239) -> (w236:bool)
        n193 = And(x="Setup.Stop on full", y=w236) -> (x .and. y?=w234:bool)
        n194 = Compound Arithmetic op=OR(w255, w237, w238, w234) -> (w227:bool)
        n195 = Not(x=w227) -> (.not. x?=w226:bool)
        n196 = And(x=w225, y=w226) -> (x .and. y?=→"Status.ScanUpdateIO":bool)
        n197 = Select(t=enum16{"Idling", "Acquiring", "Ending"}."Ending", s=w227, f=enum16{"Idling", "Acquiring", "Ending"}."Acquiring") -> (s? t:f=w250:enum16{"Idling", "Acquiring", "Ending"})
      }
      frame "Ending" {
        (unwired) FALSE ("Timed Out?")
        n198 = local read "Status.State"() -> (w336:T2)
        n199 = Equal?(x=w336, y=FPGAState."Idle") -> (x = y?=w334:bool)
        n200 = Select(t=enum16{"Idling", "Acquiring", "Ending"}."Idling", s=w334, f=enum16{"Idling", "Acquiring", "Ending"}."Ending") -> (s? t:f=w333:enum16{"Idling", "Acquiring", "Ending"})
      }
    }
    "Status.DownsampleDone" <- w208
    "Status.AcqState" <- w214
  }
  n201 = xnode "FPGA I/O Node"() -> ()  [unwired: 1 in, 2 out]
  n202 = node-c288(w7) -> ()
